vi "test Verify with Regex Scrubber Count Unique.vi"(8 "error in":errorcluster, 11 "Test Case In":refnum<class "LUnit Extensions Tests.lvclass">) -> (0 "error out":errorcluster, 3 "Test Case Out":refnum<class "LUnit Extensions Tests.lvclass">)   [LabVIEW 2020, in "LUnit Extensions Tests.lvclass"]
uses:
  LUnit Extensions Tests.lvclass
  LUnit Extensions Tests.lvclass/LUnit Extensions Tests.ctl
  240f995d-3744-484a-8956-6f48e6079b93.vi
  Source/Approval Tests/Regex Scrubber Count Unique/Regex Scrubber Count Unique.lvclass
  Source/Approval Tests/Options/Options.lvclass
  C:/Users/SAS/Desktop/ApprovalTests.LabVIEW/Source/Approval Tests/Regex Scrubber Count Unique/Regex Scrubber Count Unique.lvclass
  C:/Users/SAS/Desktop/ApprovalTests.LabVIEW/Source/Approval Tests/Scrubber/Scrubber.lvclass
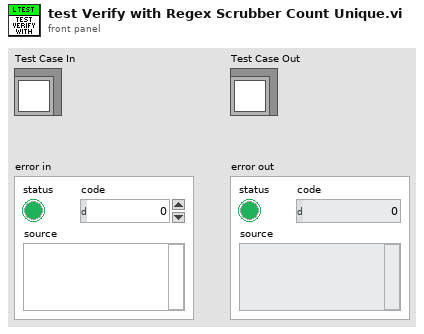
[diagram p1: front panel]
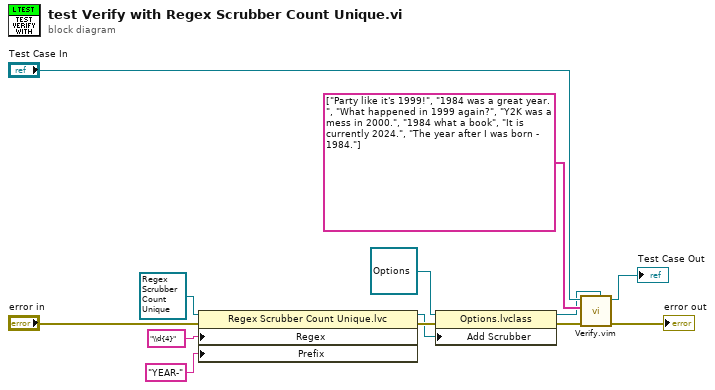
[diagram p0: block diagram]
diagram:
  n1 = property on="Property Node" class="Regex Scrubber Count Unique.lvc"(reference=refnum<class "Regex Scrubber Count Unique.lvclass"> refnum ("Approval Tests.lvlib:Regex Scrubber with Numbered Replacement.lvclass"), error in="error in", "Regex"="\\d{4}", "Prefix"="YEAR-" ("Replacement")) -> (reference out=w3:refnum<class "Regex Scrubber Count Unique.lvclass">, error out=w5:errorcluster)
  n2 = property class="Options.lvclass"(reference=refnum<class "Options.lvclass"> refnum ("Approval Tests.lvlib:Options.lvclass"), error in=w5, "Add Scrubber"=w3) -> (reference out=w2:refnum<class "Options.lvclass">, error out=w1:errorcluster)
  n3 = call "Verify.vim"("Options"=w2, "error in"=w1, "Test Data"=string[] ["Party like it's 1999!", "1984 was a great year.", "What happened in 1999 again?", "Y2K was a mess in 2000.", "1984 what a book", "It is currently 2024.", "The year after I was born - 1984."], "LUnit Test Case In"="Test Case In") -> ("error out"=→"error out":errorcluster, "LUnit Test Case Out"=→"Test Case Out":refnum<class "LUnit Extensions Tests.lvclass">)  [unwired: 6 in]
